vi "testGetViGetEvent.vi"(8 "error in (no error)":errorcluster) -> (0 "error out":errorcluster)   [LabVIEW 2018]
uses:
  src/LibReader/LibReader.lvclass
  <vilib>/addons/_JKI Toolkits/Caraya/classes/Assert/Assert Error.vi
  <vilib>/addons/_JKI Toolkits/Caraya/classes/Assert/Assert Equal Value_Variant.vi
  <vilib>/addons/_JKI Toolkits/Caraya/classes/Test/Test.lvclass
  <vilib>/addons/_JKI Toolkits/Caraya/classes/Assert/Assert.lvclass
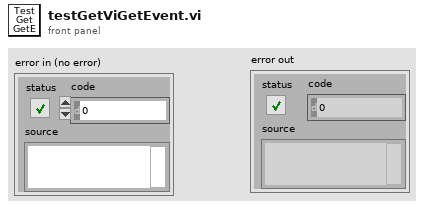
[diagram p1: front panel]
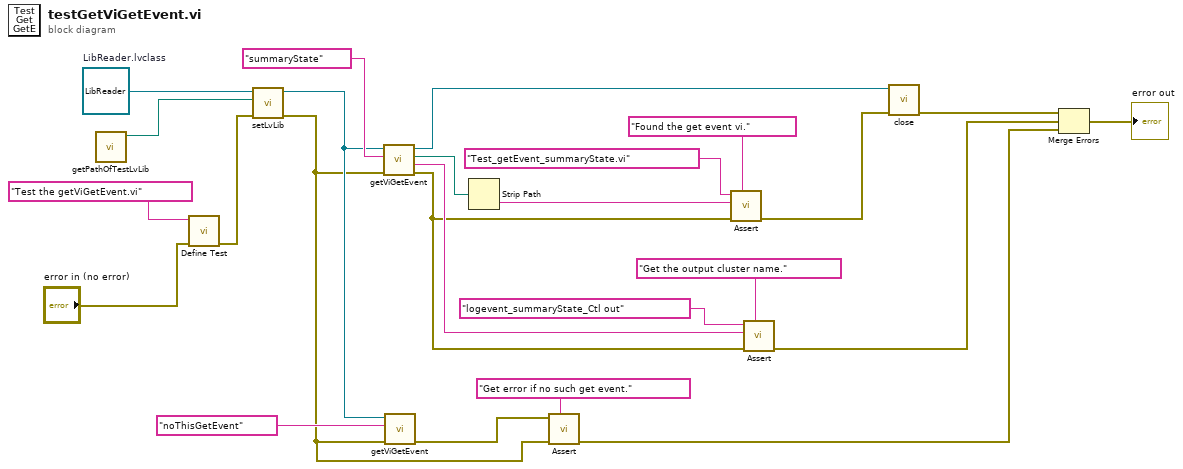
[diagram p0: block diagram]
diagram:
  w23 = refnum<class "LibReader.lvclass"> refnum  # LibReader.lvclass
  n1 = call "getPathOfTestLvLib.vi"() -> ("testLvLibPath"=w22:path)  [unwired: 11 in]
  n2 = call <vilib>:"Define Test.vi"("error in (no error)"="error in (no error)", "Label (VI Title)"="Test the getViGetEvent.vi") -> ("error out"=w21:errorcluster)  [unwired: 9 in]
  n3 = call "setLvLib.vi"("error in (no error)"=w21, "pathLvLib"=w22, "LibReader in"=w23) -> ("error out"=w9:errorcluster, "LibReader out"=w10:refnum<class "LibReader.lvclass">)  [unwired: 7 in]
  n4 = call "getViGetEvent.vi"("error in (no error)"=w9, "name"="summaryState", "LibReader in"=w10) -> ("error out"=w5:errorcluster, "clusterNameOutput"=w6:string, "pathViGetEvent"=w19:path, "LibReader out"=w20:refnum<class "LibReader.lvclass">)  [unwired: 5 in]
  n5 = call "getViGetEvent.vi"("error in (no error)"=w9, "name"="noThisGetEvent", "LibReader in"=w10) -> ("error out"=w11:errorcluster)  [unwired: 5 in, 3 out]
  n6 = Strip Path(path=w19) -> (name=w18:string)  [unwired: 1 out]
  n7 = call-poly <vilib>:"Assert.vi"("Label"="Get error if no such get event.", "error in (no error)"=w9, "Error?"=w11) -> ("error out"=w2:errorcluster)  [unwired: 8 in]
  n8 = call-poly <vilib>:"Assert.vi"("Label"="Found the get event vi.", "error in (no error)"=w5, "Y"=w18, "X"="Test_getEvent_summaryState.vi") -> ("error out"=w17:errorcluster)  [unwired: 7 in]
  n9 = call-poly <vilib>:"Assert.vi"("Label"="Get the output cluster name.", "error in (no error)"=w5, "Y"=w6, "X"="logevent_summaryState_Ctl out") -> ("error out"=w1:errorcluster)  [unwired: 7 in]
  n10 = call "close.vi"("error in (no error)"=w17, "LibReader in"=w20) -> ("error out"=w8:errorcluster)  [unwired: 8 in, 1 out]
  n11 = Merge Errors(w8, w1, w2) -> (→"error out":errorcluster)
